vi "DriveCals.vi"() -> ()   [LabVIEW 2014]
panel:
  in  "MaxStrafeIncrement":dbl=0.05
  in  "MaxDriveIncrement":dbl=0.1
  in  "ResetGyroMSAfterTurn":dbl=250.0
  in  "MaxStrafe3":dbl=0.5
  in  "MaxStrafe4":dbl=0.25
  in  "MaxStrafe2":dbl=0.75
  in  "MaxStrafe1":dbl=1.0
  in  "MaxDrivePwr3":dbl=0.5
  in  "MaxDrivePwr4":dbl=0.25
  in  "MaxDrivePwr2":dbl=0.75
  in  "MaxDrivePwr1":dbl=1.0
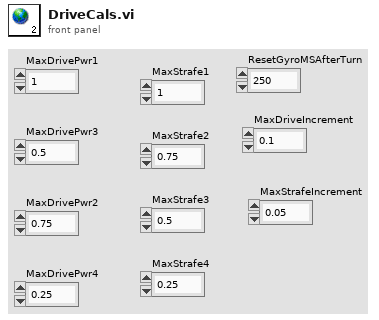
[diagram p1: front panel]
diagram:
